vi "(FPGA)servoController.vi"(10 "stop the loop":bool, 11 "pulse width (µs)":u32=2200 min=2200 max=2499) -> ()   [LabVIEW 2020]
uses:
  <vilib>/rvi/Emulation/niFpgaGetClockAttributes.vi
  <vilib>/rvi/Emulation/niFpgaSctlEmulationGetInTimedLoop.vi
  <vilib>/rvi/Emulation/niFpgaEmulationReportErrorSimple.vi
  <vilib>/rvi/eio/common/nirviEmuTemplateMethod_errors.vi
  <vilib>/rvi/Emulation/niFpgaCriticalErrorInLSC.vi
  <vilib>/eio/EIONode/EIONode.xnode
panel:
  in  "loop clock (µs) \ninput (3100 - 20000)":u32=3100 min=3100 max=20000
  out "loop clock (µs)":i16=20000
  in  "min voltage (0)":fxp<+/-,20,5>
  in  "max voltage (5)":fxp<+,5,5>=5.0
  out "current pulse width (µs)":i16
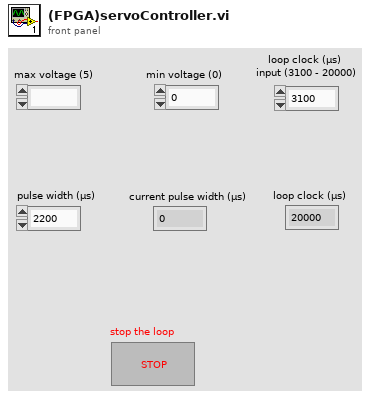
[diagram p1: front panel]
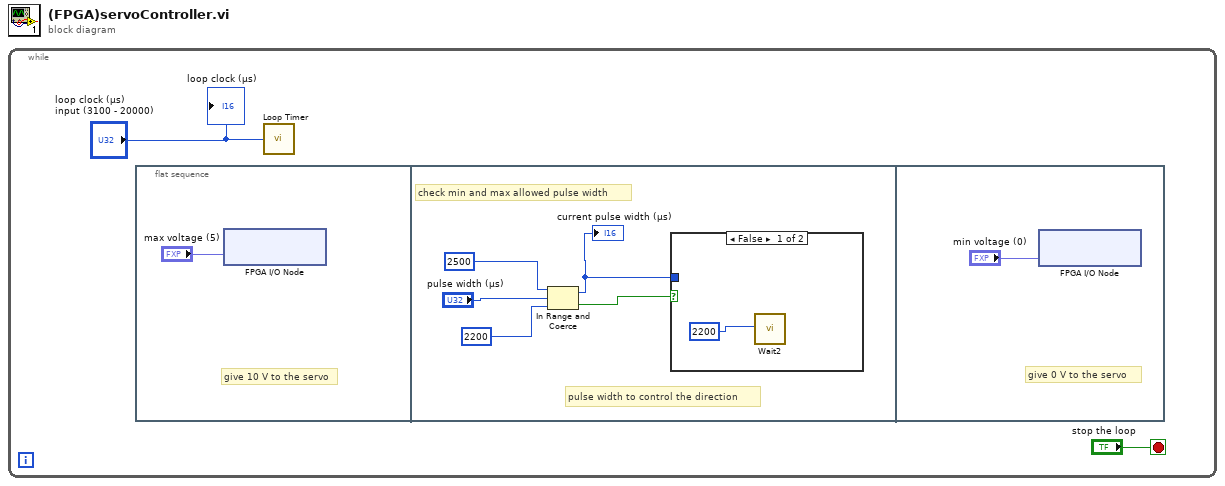
[diagram p0: block diagram]
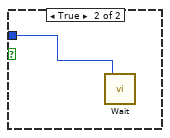
[diagram p2: hidden frame]
diagram:
  n1 = while {
    stop <- "stop the loop" stop-if-true
    n2 = flat-sequence {
      frame #0 {
        # "give 10 V to the servo"
        n3 = xnode "FPGA I/O Node"("Mod5/AO0"="max voltage (5)") -> ()  [unwired: 1 in, 1 out]
      }
      frame #1 {
        # "check min and max allowed pulse width"
        # "pulse width to control the direction"
        n4 = In Range and Coerce(upper limit=i16 2500, x="pulse width (µs)", lower limit=i16 2200) -> (coerced(x)=w4:u32, In Range?=w5:bool)
        "current pulse width (µs)" <- w4
        n5 = case shown="False" w5 {
          tunnel: w4 -> [_ w10]
          frame False {
            n6 = call "Wait2"("Count(uSec)"=i16 2200) -> ()  [unwired: 1 out]
          }
          frame True {
            n7 = call "Wait"("Count(uSec)"=w10) -> ()  [unwired: 1 out]
          }
        }
      }
      frame #2 {
        # "give 0 V to the servo"
        n8 = xnode "FPGA I/O Node"("Mod5/AO0"="min voltage (0)") -> ()  [unwired: 1 in, 1 out]
      }
    }
    n9 = call "Loop Timer"("Count(uSec)"="loop clock (µs) \ninput (3100 - 20000)") -> ()  [unwired: 1 out]
    "loop clock (µs)" <- "loop clock (µs) \ninput (3100 - 20000)"
  }
